vi "DAQ - Close.vi"() -> (0 "error out":errorcluster)   [LabVIEW 2018]
uses:
  DAQ Globals.vi
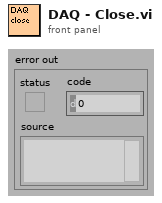
[diagram p1: front panel]
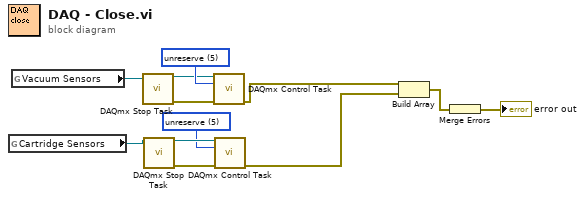
[diagram p0: block diagram]
diagram:
  w3 = 5 items=["verify"=2, "reserve"=4, "commit"=3, "unreserve"=5, "abort"=6] ("action")
  w10 = 5 items=["verify"=2, "reserve"=4, "commit"=3, "unreserve"=5, "abort"=6] ("action")
  n1 = global read "DAQ Globals.vi" "Cartridge Sensors"() -> (w2:refnum<k21>)
  n2 = global read "DAQ Globals.vi" "Vacuum Sensors"() -> (w6:refnum<k21>)
  n3 = call <vilib>:"DAQmx Stop Task.vi"("task/channels in"=w6) -> ("task out"=w9:refnum<k21>, "error out"=w8:errorcluster)  [unwired: 13 in]
  n4 = call <vilib>:"DAQmx Stop Task.vi"("task/channels in"=w2) -> ("task out"=w4:refnum<k21>, "error out"=w5:errorcluster)  [unwired: 13 in]
  n5 = call <vilib>:"DAQmx Control Task.vi"("task/channels in"=w9, "action"=w10, "error in"=w8) -> ("error out"=w7:errorcluster)  [unwired: 11 in, 1 out]
  n6 = call <vilib>:"DAQmx Control Task.vi"("task/channels in"=w4, "action"=w3, "error in"=w5) -> ("error out"=w1:errorcluster)  [unwired: 11 in, 1 out]
  n7 = Build Array(w7, w1) -> (w11:errorcluster[])
  n8 = Merge Errors(w11) -> (→"error out":errorcluster)
